vi "DELETE Sample Rate.vi"   [LabVIEW 2013]
uses:
  Action.ctl
  Power Peak Calibration Input FGV Selector.ctl
types:
  T1 = typedef "Power Peak Calibration Input FGV Selector.ctl" = enum16{"Samples/Sweep", "Num Sweeps", "Sample Rate"}
  T2 = typedef "Action.ctl" = enum16{"GET", "PUT", "DELETE"}
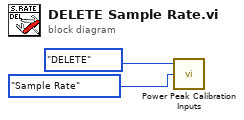
[diagram p0: block diagram]
diagram:
  n1 = call "Power Peak Calibration Inputs.vi"("Calibration Input FGV Selector"=Power_Peak_Calibration_Input_FGV_Selector."Sample Rate", "Verb"=Action."DELETE") -> ()  [unwired: 1 in, 1 out]
